vi "start_movie.vi"(8 "error in (no error)":errorcluster, 10 "frames per second":dbl, 11 "DataCollectionDL091104Scaffold in":refnum<class "DataCollectionDL091104Scaffold.lvclass">) -> (0 "error out":errorcluster, 3 "DataCollectionDL091104Scaffold out":refnum<class "DataCollectionDL091104Scaffold.lvclass">)   [LabVIEW 2010, in "DataCollectionDL091104Scaffold.lvclass"]
uses:
  DataCollectionDL091104Scaffold.lvclass
  DataCollectionDL091104Scaffold.lvclass/DataCollectionDL091104Scaffold.ctl
  common/classes/ErrorController/ErrorController/class_data.vi
  common/classes/ErrorController/ErrorController/ErrorController.lvclass
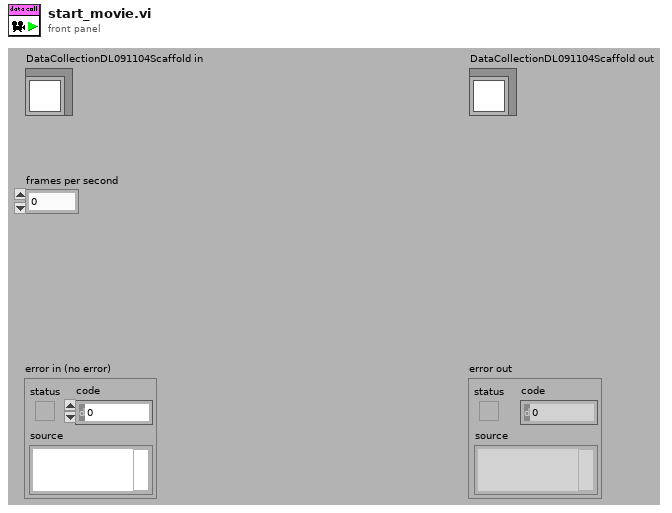
[diagram p1: front panel]
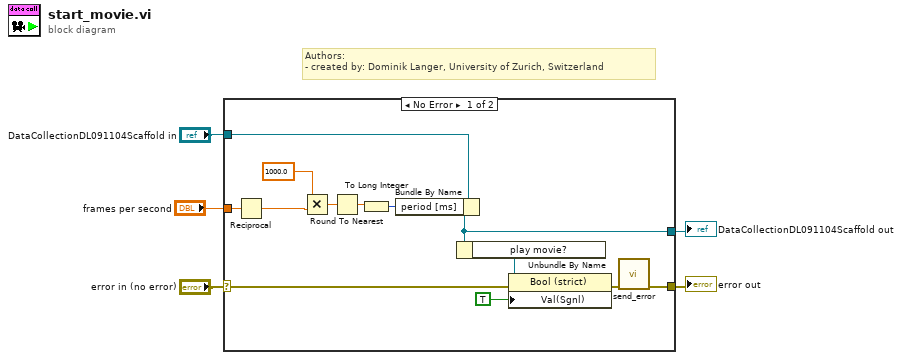
[diagram p0: block diagram]
diagram:
  # "Authors: \n- created by: Dominik Langer, University of Zurich, Switzerland"
  n1 = case shown="No Error" "error in (no error)" {
    selector: "error in (no error)" -> [w18 w20]
    tunnel: [w6 w20] -> w4
    tunnel: [w14 w19] -> w2
    tunnel: "DataCollectionDL091104Scaffold in" -> [w15 w19]
    tunnel: "frames per second" -> [w13 _]
    frame No Error {
      n2 = Reciprocal(x=w13) -> (1/x=w8:dbl)
      n3 = Multiply(x=1000.0, y=w8) -> (x*y=w11:dbl)
      n4 = Round To Nearest(number=w11) -> (nearest integer value=w10:dbl)
      n5 = To Long Integer(number=w10) -> (32bit integer=w9:i32)
      n6 = Bundle By Name(cluster=w15, "period [ms]"=w9) -> (w14:refnum<class "DataCollectionDL091104Scaffold.lvclass">)
      n7 = Unbundle By Name(w14) -> ("play movie?"=w17:refnum<vi>)
      n8 = property class="Bool (strict)"(reference=w17, error in=w18, "Val(Sgnl)"=TRUE) -> (error out=w7:errorcluster)  [unwired: 1 out]
      n9 = call "send_error.vi"("error in (no error)"=w7) -> ("error out"=w6:errorcluster)  [unwired: 10 in]
    }
    frame Error {
    }
  }
  "error out" <- w4
  "DataCollectionDL091104Scaffold out" <- w2
